vi "AT Set Enum Index A.vi"(8 "error in (no error)":errorcluster, 9 "Value":i32, 10 "Feature":string, 11 "Handle":i32) -> (0 "error out":errorcluster, 3 "Status":i32)   [LabVIEW 2009]
doc: "Set Enum Index\n\nOutput:\n I32 Status\n\nInput:\n I32 Handle\n String Feature\n I32 Value\n\nThis function sets the currently selected index of the specified enumerated feature. The index is zero based and should be in the range 0 to Count-1, where Count has been retrieved using the GetEnumCount function. An error will be returned if the feature is read only, currently not writable, the index is outside the allowed range, not an enumerated feature, or the feature is not implemented by the camera. In some cases an index within the range may not be allowed if its availability depends on other features values, in this case an error will be returned if this index is applied."
uses:
  atcoreA.dll
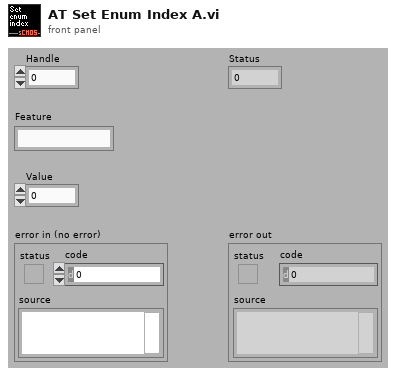
[diagram p1: front panel]
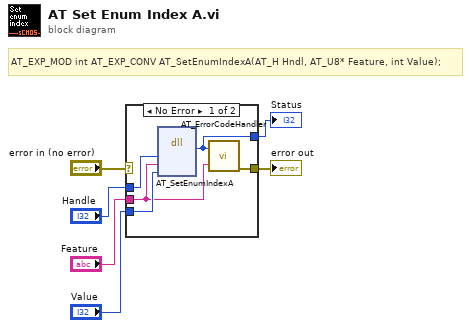
[diagram p0: block diagram]
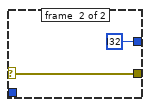
[diagram p2: hidden frame]
diagram:
  # "AT_EXP_MOD int AT_EXP_CONV AT_SetEnumIndexA(AT_H Hndl, AT_U8* Feature, int Value);"
  n1 = case shown="No Error" "error in (no error)" {
    selector: "error in (no error)" -> [_ w13]
    tunnel: [w7 i32 ? ("return type")] -> w6
    tunnel: "Handle" -> [w11 _]
    tunnel: "Feature" -> [w8 _]
    tunnel: "Value" -> [w10 _]
    tunnel: [w9 w13] -> w2
    frame #0 {
      n2 = dll-call lib="atcoreA.dll" fn="AT_SetEnumIndexA"("Handle"=w11, "Feature"=w8, "Value"=w10) -> ("Status"=w7:i32)  [unwired: 6 in, 2 out]
      n3 = call "AT_ErrorCodeHandler.vi"("Error"=w7, "Feature Name"=w8) -> ("error out"=w9:errorcluster)  [unwired: 5 in]
    }
    frame #1 {
    }
  }
  "Status" <- w6
  "error out" <- w2
